vi "RangeI2C-loopFast.vi"(0 "Remote IP Address":string="192.168.124.53", 1 "Remote Port":u16=502, 2 "I2C Operation Control":T1(ring)=enum."Command Find Range", 3 "SCL DIO Ch. No.":u16=2, 4 "SDA DIO Ch. No.":u16=3, 5 "Current Address":u8=216 min=202 max=224 step=2, 8 "New Address":u8=224 min=202 max=224 step=2) -> (6 "Range (cm)":dbl=-102.0, 7 "Range (in.)":dbl=-40.15748031496063 format="%#.2g")   [LabVIEW 2022 SP3]
panel:
  in  "Clear Graph":bool
  in  "Zero (cm)":dbl
  out "Waveform Graph":dbl[](graph)=[-101.0, -101.0, -101.0, -101.0, -102.0, -102.0, -102.0, -102.0, -102.0, -102.0, -102.0, -102.0, -102.0, -102.0, -102.0, -102.0, -102.0, -102.0, -102.0, -102.0, -102.0, -102.0, -102.0, -102.0, -102.0, -102.0, -102.0, -102.0, -102.0, -102.0, -102.0, -102.0, -102.0, -102.0, -102.0, -102.0, -102.0, -102.0, -102.0, -102.0, -102.0, -102.0, -102.0, -102.0, -102.0, -102.0, -102.0, -102.0, -102.0]
  in  "stop":bool
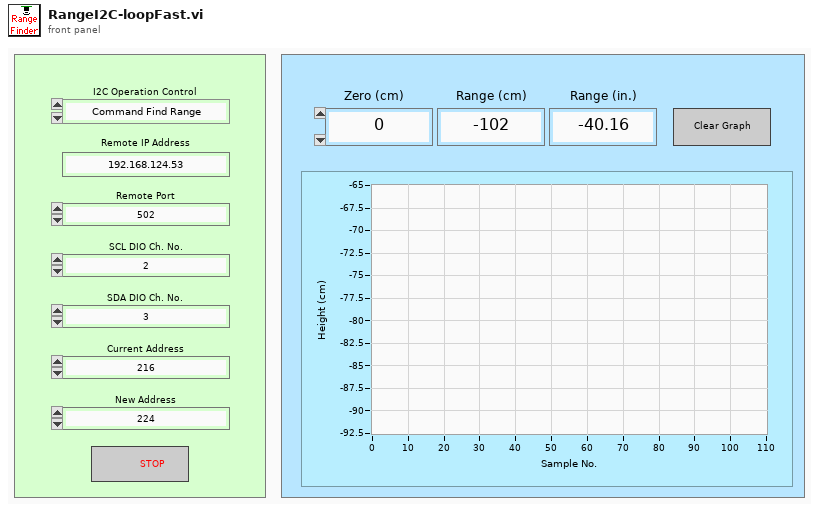
[diagram p1: front panel]
types:
  T1 = enum16{"Configure I2C Settings", "Command Find Range", "Command Read Range", "Report the last range value", "Change sensor address", "Wait to range 100ms"}
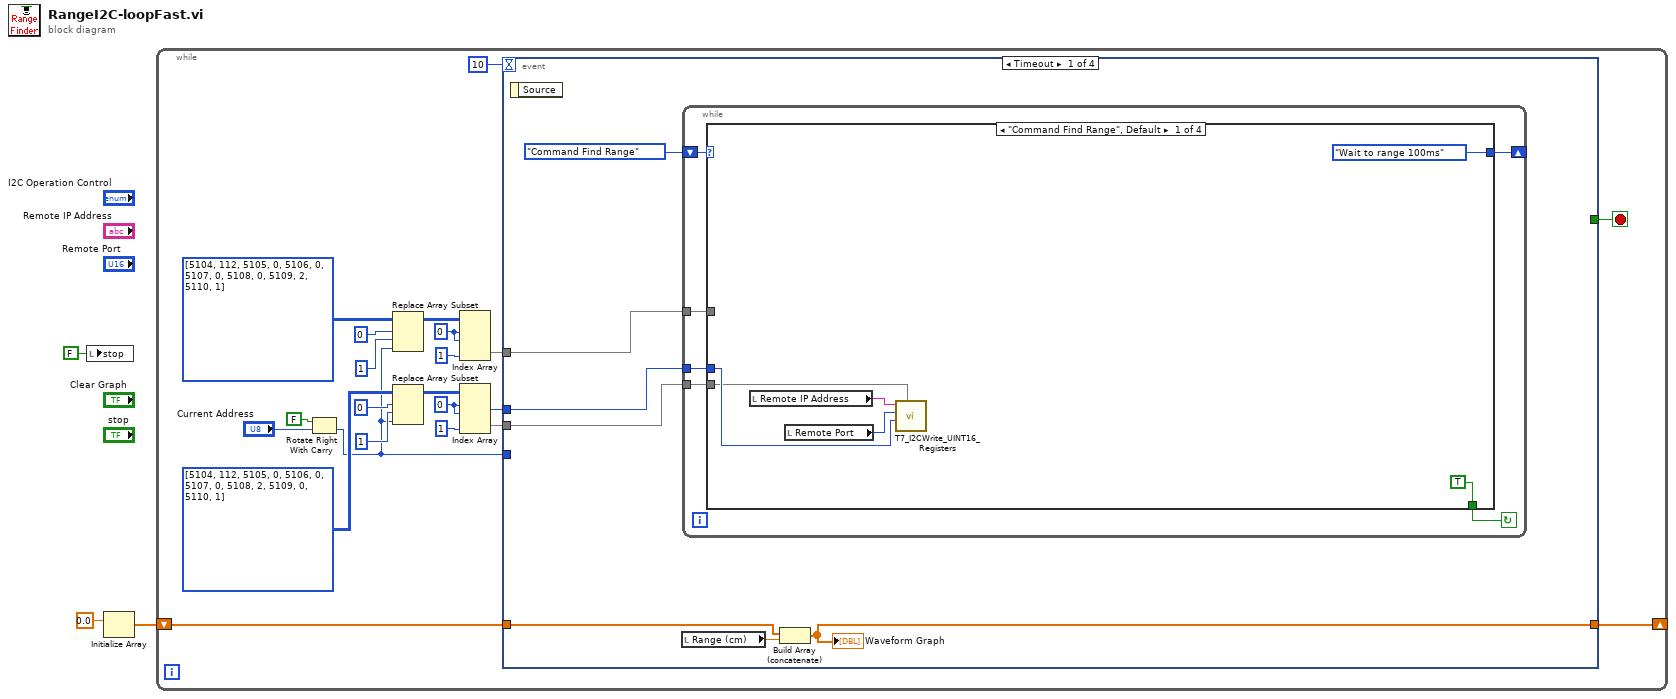
[diagram p0: block diagram]
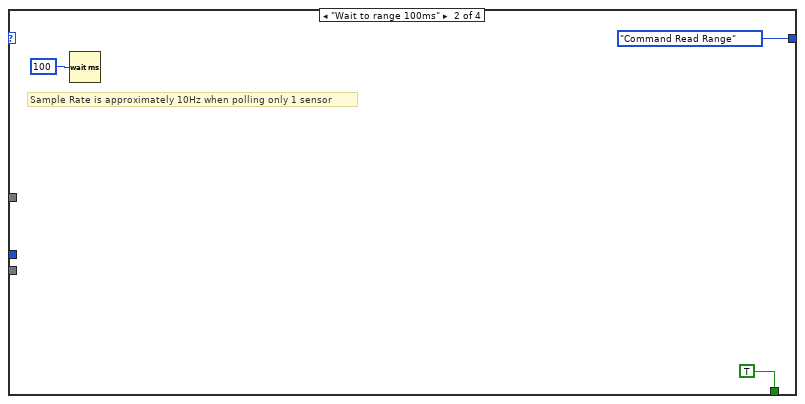
[diagram p2: hidden frame]
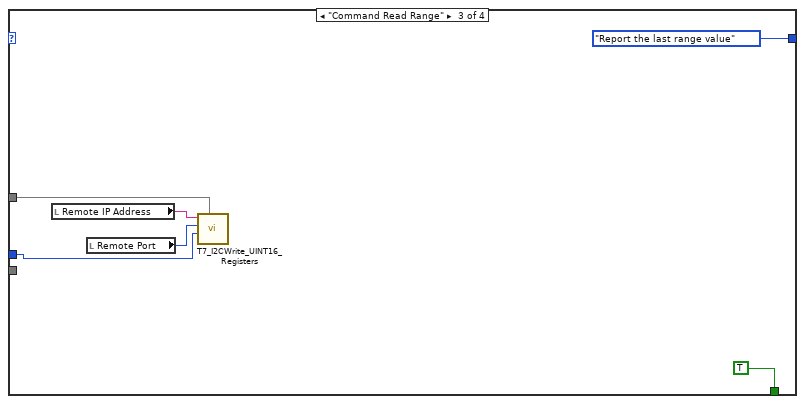
[diagram p3: hidden frame]
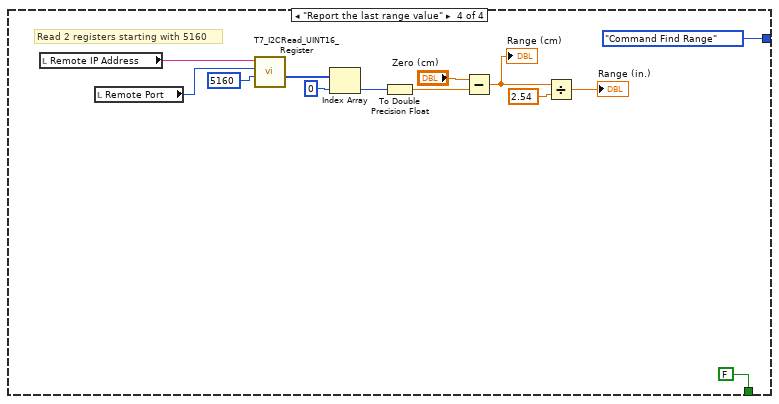
[diagram p4: hidden frame]
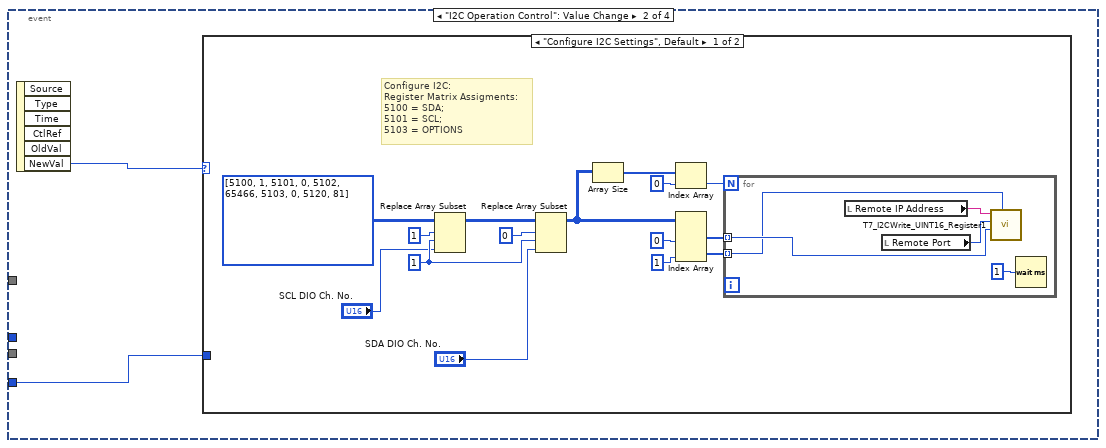
[diagram p5: hidden frame]
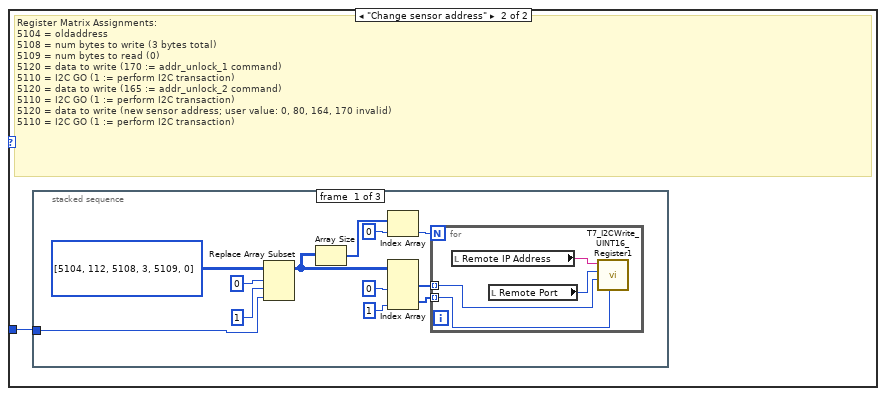
[diagram p6: hidden frame]
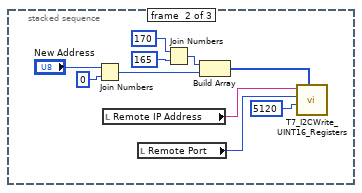
[diagram p7: hidden frame]
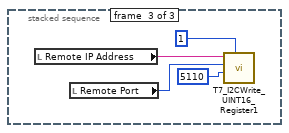
[diagram p8: hidden frame]
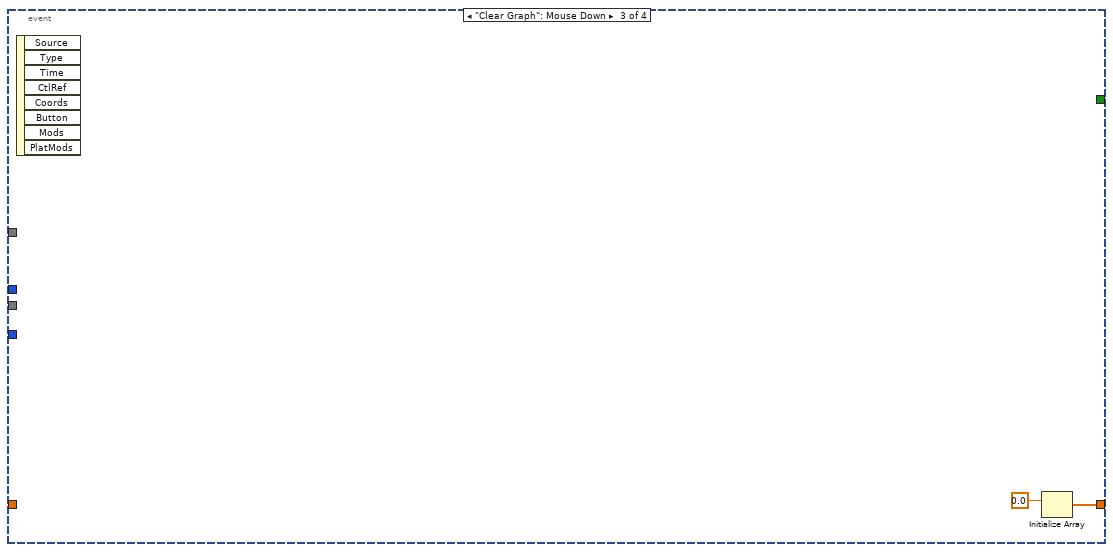
[diagram p9: hidden frame]
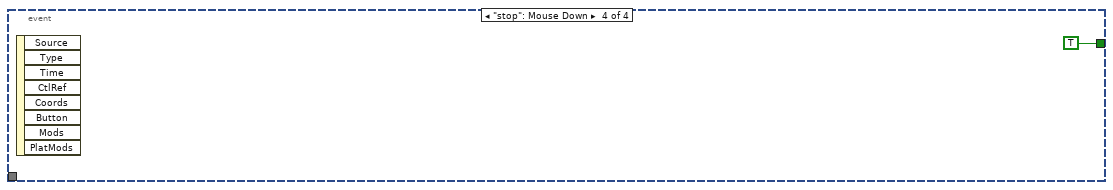
[diagram p10: hidden frame]
diagram:
  n1 = local write "stop"(FALSE ("stop")) -> ()
  n2 = Initialize Array(0.0 ("element")) -> (w3:dbl[])  [unwired: 1 in]
  n3 = while {
    shift-right: [w24] -> _
    shift-left: w3 -> [w23]
    stop <- w25 stop-if-true
    w13 = 0 ("disabled index (col)")
    w14 = 0 ("disabled index (col)")
    n4 = Rotate Right With Carry(2:"Current Address", 3:FALSE ("carry")) -> (0:w7:u8)  [unwired: 1 out]
    n5 = Replace Array Subset(array=i32[][] [[5104, 112], [5105, 0], [5106, 0], [5107, 0], [5108, 0], [5109, 2], [5110, 1]], new element=w7, index (row)=0, index (col)=1 ("disabled index (col)")) -> (w12:i32[][])
    n6 = Replace Array Subset(array=i32[][] [[5104, 112], [5105, 0], [5106, 0], [5107, 0], [5108, 2], [5109, 0], [5110, 1]], new element=w7, index (row)=0, index (col)=1 ("disabled index (col)")) -> (w19:i32[][])
    n7 = Index Array(array=w12, index (row) #1=w13, index (col) #1=w13, index (col) #2=1 ("index (col)")) -> (element #2=w6:i32[])  [unwired: 1 in, 1 out]
    n8 = Index Array(array=w19, index (row) #1=w14, index (col) #1=w14, index (col) #2=1 ("index (col)")) -> (element #1=w4:i32, element #2=w5:i32[])  [unwired: 1 in]
    n9 = event shown="[0] Timeout" {
      selector: _ -> [_ _ _ _]
      dyn-events: _ -> [_ _ _ _]
      timeout: 10 -> [_ _ _ _]
      tunnel: [_ _ _ TRUE] -> w25
      tunnel: [w31 _ w120 _] -> w24
      tunnel: w23 -> [w30 _ _ _]
      tunnel: w7 -> [_ w67 _ _]
      tunnel: w6 -> [w29 _ _ _]
      tunnel: w5 -> [w28 _ _ _]
      tunnel: w4 -> [w27 _ _ _]
      event Timeout {
        n10 = event-data() -> ()  [unwired: 1 in, 1 out]
        n11 = local read "Range (cm)"() -> (w32:dbl)
        n12 = while {
          tunnel: w29 -> [w36]
          tunnel: w28 -> [w35]
          tunnel: w27 -> [w34]
          shift-right: [w38] -> _
          shift-left: T1."Command Find Range" ("I2C Operation Control") -> [w37]
          stop <- w33 continue-if-true
          n13 = case shown="\"Command Find Range\", Default" w37 {
            tunnel: [T1."Wait to range 100ms" ("I2C Operation Control") T1."Command Read Range" ("I2C Operation Control") T1."Report the last range value" ("I2C Operation Control") T1."Command Find Range" ("I2C Operation Control")] -> w38
            tunnel: w34 -> [w43 _ w49 _]
            tunnel: w35 -> [w42 _ _ _]
            tunnel: w36 -> [_ _ w50 _]
            tunnel: [TRUE TRUE TRUE FALSE] -> w33
            frame "Command Find Range", Default {
              n14 = local read "Remote IP Address"() -> (w41:string)
              n15 = local read "Remote Port"() -> (w40:u16)
              n16 = call "T7_I2CWrite_UINT16_Registers.vi"("Remote IP Address"=w41, "Remote Port"=w40, "Starting Address"=w43, "UINT16 to Write"=w42) -> ()  [unwired: 5 in, 2 out]
            }
            frame "Wait to range 100ms" {
              # "Sample Rate is approximately 10Hz when polling only 1 sensor"
              n17 = Wait (ms)(milliseconds to wait=u32 100) -> ()  [unwired: 1 out]
            }
            frame "Command Read Range" {
              n18 = local read "Remote IP Address"() -> (w52:string)
              n19 = local read "Remote Port"() -> (w51:u16)
              n20 = call "T7_I2CWrite_UINT16_Registers.vi"("Remote IP Address"=w52, "Remote Port"=w51, "Starting Address"=w49, "UINT16 to Write"=w50) -> ()  [unwired: 5 in, 2 out]
            }
            frame "Report the last range value" {
              # "Read 2 registers starting with 5160"
              n21 = local read "Remote IP Address"() -> (w64:string)
              n22 = local read "Remote Port"() -> (w65:u16)
              n23 = call "T7_I2CRead_UINT16_Register.vi"("FirstChannel"=5160, "Remote Port"=w65, "Remote IP Address"=w64) -> ("Raw Data Read"=w63:u16[])  [unwired: 6 in, 2 out]
              n24 = Index Array(array=w63, index=0) -> (element=w61:u16)
              n25 = To Double Precision Float(number=w61) -> (double precision float=w55:dbl)
              n26 = Subtract(x="Zero (cm)", y=w55) -> (x-y=w57:dbl)
              "Range (cm)" <- w57
              n27 = Divide(x=w57, y=2.54) -> (x/y=→"Range (in.)":dbl)
            }
          }
        }
        n28 = Build Array (concatenate)(w30, w32) -> (w31:dbl[])
        "Waveform Graph" <- w31
      }
      event "I2C Operation Control": Value Change {
        n29 = event-data() -> ("NewVal"=w68:T1)  [unwired: 1 in, 5 out]
        n30 = case shown="\"Configure I2C Settings\", Default" w68 {
          tunnel: w67 -> [_ w89]
          frame "Configure I2C Settings", Default {
            w73 = 1 ("disabled index (col)")
            # "Configure I2C: \nRegister Matrix Assigments:\n5100 = SDA;\n5101 = SCL;\n5103 = OPTIONS"
            n31 = Replace Array Subset(array=i32[][] [[5100, 1], [5101, 0], [5102, 65466], [5103, 0], [5120, 81]], new element="SCL DIO Ch. No.", index (row)=1, index (col)=w73) -> (w72:i32[][])
            n32 = Replace Array Subset(array=w72, new element="SDA DIO Ch. No.", index (row)=0, index (col)=w73) -> (w69:i32[][])
            n33 = Array Size(array=w69) -> (size(s)=w83:i32[])
            n34 = Index Array(array=w83, index=0) -> (element=w81:i32)
            n35 = Index Array(array=w69, index (col) #1=0 ("disabled index (col)"), index (col) #2=1 ("index (col)")) -> (element #1=w78:i32[], element #2=w77:i32[])  [unwired: 2 in]
            n36 = for {
              N: w81 -> [_]
              tunnel: w78 -> [w88] mode=indexing
              tunnel: w77 -> [w87] mode=indexing
              n37 = local read "Remote IP Address"() -> (w86:string)
              n38 = local read "Remote Port"() -> (w85:u16)
              n39 = call "T7_I2CWrite_UINT16_Register1.vi"("Remote IP Address"=w86, "Remote Port"=w85, "Starting Address"=w88, "UINT16 to Write"=w87) -> ()  [unwired: 5 in, 2 out]
              n40 = Wait (ms)(milliseconds to wait=u32 1) -> ()  [unwired: 1 out]
            }
          }
          frame "Change sensor address" {
            # "Register Matrix Assignments:\n5104 = oldaddress\n5108 = num bytes to write (3 bytes total)\n5109 = num bytes to read (0)\n5120 = data to write (170 := addr_unlock_1 command)\n5110 = I2C GO (1 := perform I2C transaction)\n5120 = data to write (165 := addr_unlock_2 command)\n5110 = I2C GO (1 := perform I2C transaction)\n5120 = data to write (new sensor address; user value: 0, 80, 164, 170 invalid)\n5110 = I2C GO (1 := perform I2C transaction)"
            n41 = stacked-sequence {
              tunnel: w89 -> [w92 _ _]
              frame #0 {
                n42 = Replace Array Subset(array=i32[][] [[5104, 112], [5108, 3], [5109, 0]], new element=w92, index (row)=0, index (col)=1 ("disabled index (col)")) -> (w90:i32[][])
                n43 = Array Size(array=w90) -> (size(s)=w101:i32[])
                n44 = Index Array(array=w101, index=0) -> (element=w99:i32)
                n45 = Index Array(array=w90, index (col) #1=0 ("disabled index (col)"), index (col) #2=1 ("index (col)")) -> (element #1=w96:i32[], element #2=w95:i32[])  [unwired: 2 in]
                n46 = for {
                  N: w99 -> [_]
                  tunnel: w96 -> [w105] mode=indexing
                  tunnel: w95 -> [w104] mode=indexing
                  n47 = local read "Remote IP Address"() -> (w103:string)
                  n48 = local read "Remote Port"() -> (w102:u16)
                  n49 = call "T7_I2CWrite_UINT16_Register1.vi"("Remote IP Address"=w103, "Remote Port"=w102, "Starting Address"=w105, "UINT16 to Write"=w104) -> ()  [unwired: 5 in, 2 out]
                }
              }
              frame #1 {
                n50 = Join Numbers(hi="New Address", lo=u8 0) -> ((hi.lo)=w110:u16)
                n51 = local read "Remote IP Address"() -> (w108:string)
                n52 = local read "Remote Port"() -> (w107:u16)
                n53 = Join Numbers(hi=u8 170, lo=u8 165) -> ((hi.lo)=w111:u16)
                n54 = Build Array(w111, w110) -> (w109:u16[])
                n55 = call "T7_I2CWrite_UINT16_Registers.vi"("Remote IP Address"=w108, "Remote Port"=w107, "Starting Address"=u16 5120, "UINT16 to Write"=w109) -> ()  [unwired: 5 in, 2 out]
              }
              frame #2 {
                n56 = local read "Remote IP Address"() -> (w117:string)
                n57 = local read "Remote Port"() -> (w116:u16)
                n58 = call "T7_I2CWrite_UINT16_Register1.vi"("Remote IP Address"=w117, "Remote Port"=w116, "Starting Address"=u16 5110, "UINT16 to Write"=u16 1) -> ()  [unwired: 5 in, 2 out]
              }
            }
          }
        }
      }
      event "Clear Graph": Mouse Down {
        n59 = event-data() -> ()  [unwired: 1 in, 8 out]
        n60 = Initialize Array(0.0 ("element")) -> (w120:dbl[])  [unwired: 1 in]
      }
      event "stop": Mouse Down {
        n61 = event-data() -> ()  [unwired: 1 in, 8 out]
      }
    }
  }
